vi "GUNSC_LibIsEnabled.vi"(8 "error in (no error)":errorcluster) -> (0 "error out":errorcluster, 2 "enabled":bool)   [LabVIEW 2014]
uses:
  public/c/lib/libunsc.so
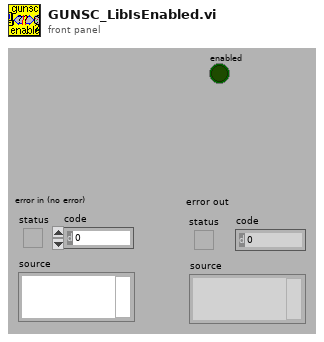
[diagram p1: front panel]
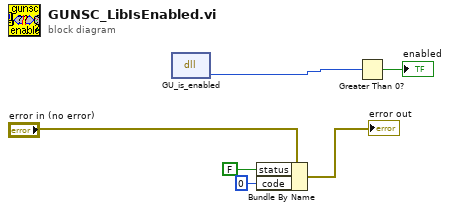
[diagram p0: block diagram]
diagram:
  n1 = dll-call lib="home/sispi/Panview-1.13.0-64b/PAN/Modules/GUNSC/public/c/lib/libunsc.so" fn="GU_is_enabled"() -> ("return type"=w6:i32)  [unwired: 3 in, 2 out]
  n2 = Bundle By Name(cluster="error in (no error)", "status"=FALSE, "code"=0) -> (→"error out":errorcluster)
  n3 = Greater Than 0?(x=w6) -> (x > 0?=→"enabled":bool)
